vi "QBrush.vi"(8 "Error In":errorcluster, 9 "brushStyle (SolidPattern)":T1=1 items=["NoBrush"=0, "SolidPattern"=1, "Dense1Pattern"=2, "Dense2Pattern"=3, "Dense3Pattern"=4, "Dense4Pattern"=5, "Dense5Pattern"=6, "Dense6Pattern"=7, "Dense7Pattern"=8, "HorPattern"=9, "VerPattern"=10, "CrossPattern"=11, "BDiagPattern"=12, "FDiagPattern"=13, "DiagCrossPattern"=14, "LinearGradientPattern"=15, "RadialGradientPattern"=16, "ConicalGradientPattern"=17, "TexturePattern"=24], 10 "color":u32(colorbox)) -> (0 "Error Out":errorcluster, 3 "New QBrush":refnum<class "QBrush.lvclass">)   [LabVIEW 2014, in "QBrush.lvclass"]
doc: "LabVIEW-specific documentation is not yet available. See <b>https://doc.qt.io/qt-5/qbrush.html#QBrush</b>"
uses:
  QBrush.lvclass
  LQ Core/Qt/BrushStyle.ctl
  LQ Core/LQSerialData/LQSerialData.lvclass/LQSerialData.ctl
  LQ Core/LQ Core.lvlib
  LQ Core/LQSerialData/LQSerialData.lvclass
  LQ Core/Qt/Qt.lvlib
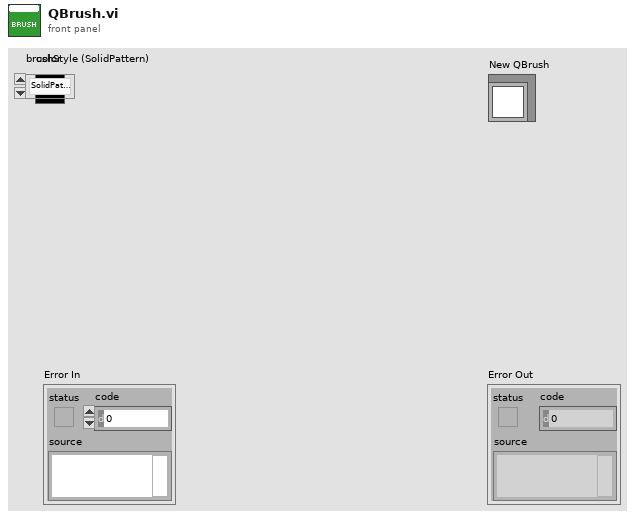
[diagram p1: front panel]
types:
  T1 = typedef "Qt.lvlib/BrushStyle.ctl" = i32
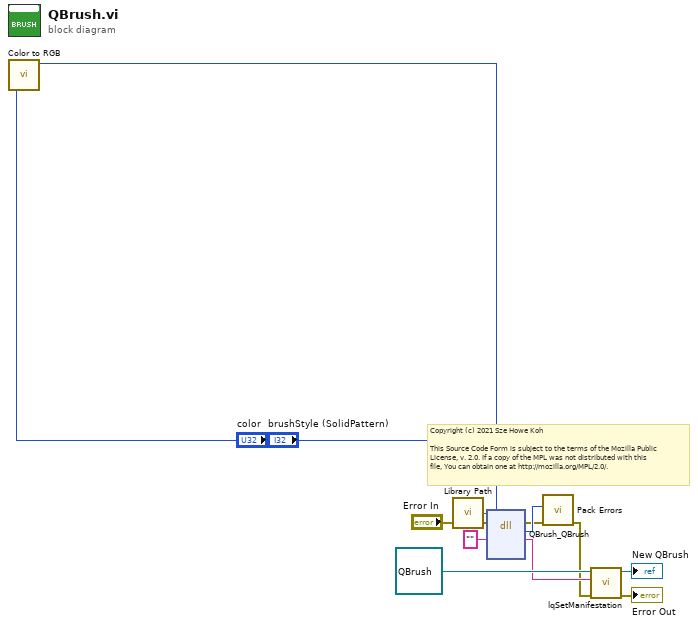
[diagram p0: block diagram]
diagram:
  # "Copyright (c) 2021 Sze Howe Koh\n\nThis Source Code Form is subject to the terms of the Mozilla Public\nLicense, v. 2.0. If a copy of the MPL was not distributed with this\nfile, You can obtain one at http://mozilla.org/MPL/2.0/."
  n1 = call <vilib>:"Color to RGB.vi"("Color"="color") -> ("Resolved Color"=w2:u32)  [unwired: 3 out]
  n2 = call "Library Path.vi"() -> ("Library Path"=w8:path)
  n3 = dll-call lib="?" fn="QBrush_QBrush"(path in=w8, error in="Error In", "_retVal"="", "color"=w2, "brushStyle"="brushStyle (SolidPattern)") -> (error out=w6:errorcluster, w7:i32, "_retVal"=w9:string)  [unwired: 3 in, 1 out]
  n4 = call "Pack Errors.vi"("Error In"=w6, "Error Code"=w7) -> ("Error Out"=w5:errorcluster)  [unwired: 9 in]
  n5 = call "lqSetManifestation.vi"("Error In"=w5, "Manifestation"=w9, "LQSerialData in"=refnum<class "QBrush.lvclass"> refnum ("QBrush")) -> ("Error Out"=→"Error Out":errorcluster, "LQSerialData out"=→"New QBrush":refnum<class "QBrush.lvclass">)  [unwired: 7 in]
